vi "Omniax_mDrive_Zonly_2019EPICS.vi"() -> ()   [LabVIEW 2015]
uses:
  <vilib>/Utility/file.llb/Read From Spreadsheet File (I64).vi
  <vilib>/Utility/file.llb/Read From Spreadsheet File (string).vi
  <userlib>/caLab/Private/Put_DBL_PV.vi
  <vilib>/Instr/_visa.llb/VISA Configure Serial Port (Instr).vi
  <userlib>/caLab/Private/Get_PV.vi
  <userlib>/caLab/Private/Put_DBL-1D_PV-1D.vi
  <userlib>/caLab/Private/Get_PV-1D.vi
  <vilib>/Utility/file.llb/Write To Spreadsheet File (I64).vi
panel:
  out "x = y?":bool
  out "EPICS RQs":dbl[][](array[numeric])
  out "Status":bool
  in  "Pressure Overide":bool
  in  "Crash Override":bool
  in  "Open?":bool
  in  "Facing up?":bool
  in  "Heater retracted?":bool
  out "APX:MZ_MVG":bool
  out "inside HPC?":bool
  out "HPC01<0.001?":bool
  out "APX:V5 opened?":bool
  out "Isolated from GND?":bool
  out "APX:MZ_LIM":bool
  out "APX:MZ_RDY":bool
  in  "APX:MZ_RQ":dbl=10.0 min=10.0 max=60.0 step=0.1 format="%_6g"
  in  "APX:MZ_VLC_RQ":dbl=0.40000000000000013 min=0.1 max=0.61 step=0.1
  out "Z Velocity SP step/sec":i32=102400 min=1 max=153600
  out "Z Step SP":i32=-20000 min=0 max=102400000 step=500
  out "Z Step PV":i32 max=2000
  out "Dev5 Voltage":dbl
  out "Z max step":i32
  in  "V5 position 15360000":i32
  out "APX:MZ_VLC_PV":dbl format="%.3f"
  out "Presets":i32[][](array[numeric])
  in  "stop":bool
  in  "Tab Control 3":enum32{"Console", "Reset", "Bypass"}(tab)
  out "APX:MZ status":string="Cancel"
  out "Status Message":string="HP cell pressure too high! or "
  in  "Reset Z Position mm":dbl
  out "Reset Z Motor Steps":i32
  in  "Reset":bool
  out "Z Position MV mm":dbl
  in  "Clear ZY":bool
  out "R Backlash steps/sec":i32
  out "R Backlash":i32
  out "R Holding Current %":i32
  out "R Run Current %":i32
  out "R offset deg":dbl
  out "R deg/rev":dbl
  out "R steps/rev":u32
  out "R velocity PV step/sec":i32
  out "Z COM PORT":refnum<visa-resource-name>="COM5"
  out "Z Backlash steps/sec":i32
  out "Z Backlash":i32
  out "Z Holding Current %":i32
  out "Z Run Current %":i32
  out "Z offset mm":dbl
  out "Z mm/rev":dbl
  out "Z steps/rev":u32
  out "Z  velocity PV step/sec":i32=102400
  out "Z MINPOS":i32=-94296
  out "Z MAXPOS":i32=-34296
  out "APX:MZ_PV":dbl format="%_5g"
  out "X velocity PV step/sec":i32
  out "X Backlash steps/sec":i32
  out "X Backlash":i32
  out "X Holding Current %":i32
  out "X Run Current %":i32
  out "X offset mm":dbl
  out "X mm/rev":dbl
  out "X steps/rev":u32
  out "Y Backlash steps/sec":i32
  out "Y Backlash":i32
  out "Y Holding Current %":i32
  out "Y Run Current %":i32
  out "Y offset mm":dbl
  out "Y mm/rev":dbl
  out "Y steps/rev":u32
  out "Y velocity PV step/sec":i32
  in  "APX:MXYZR_STOP":bool
  # "COM14"
  # "APX:MZ"
  # "355.7"
  # "345"
  # "20 degree"
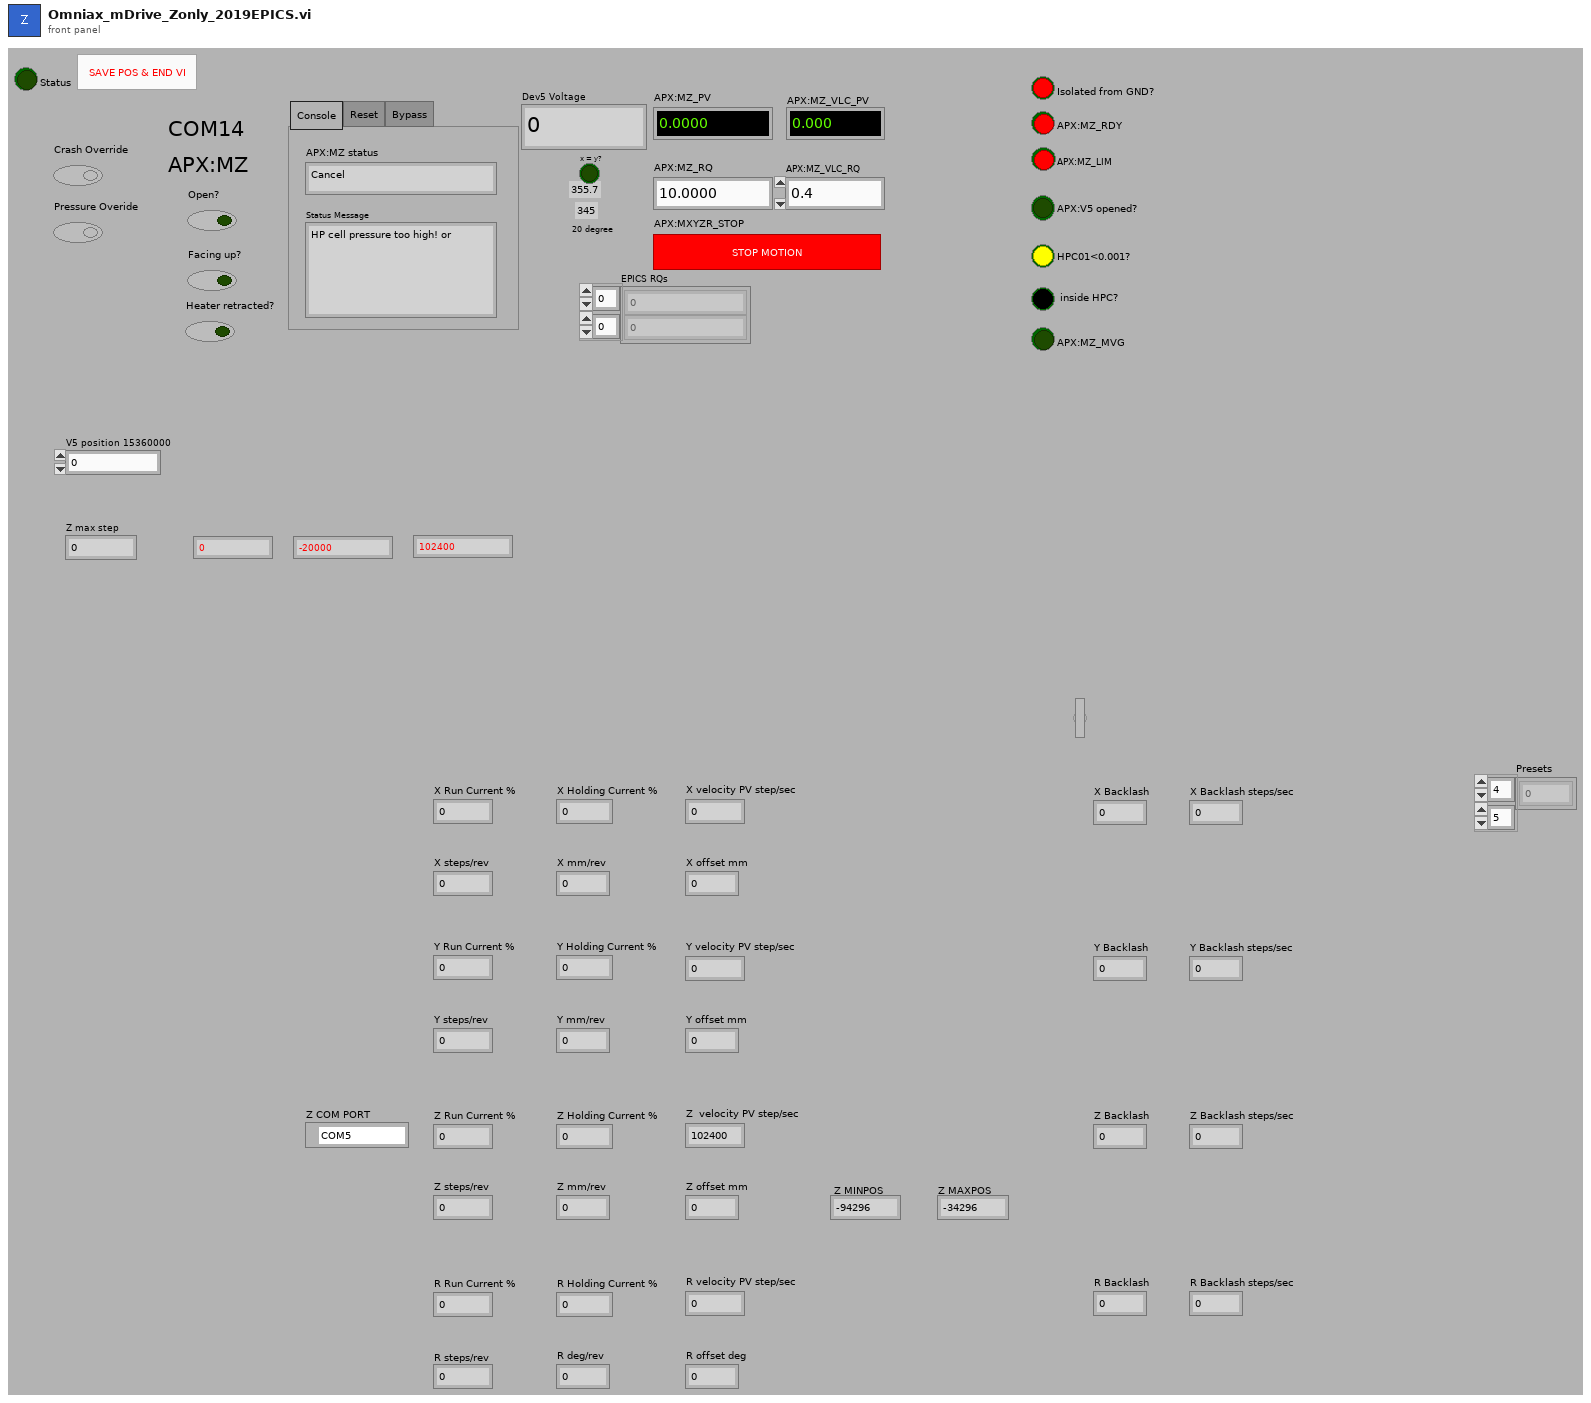
[diagram p1: front panel]
types:
  T1 = enum16{"Stop", "Reset", "Run Current", "Holding Current", "Accel Rate", "Decel Rate", "Move to Relative Position", "Move to Absolute Position", "Echo Mode", "Print Parameter", "Send String", "Microstep Resolution", "Set Current Position", "Max Velocity"}
  T2 = enum8{"Enabled", "Disabled", "Disabled and Grayed Out"}
  T3 = cluster{"first row[0]":i64, "first row[1]":i64, "first row[2]":i64, "first row[3]":i64, "first row[4]":i64, "first row[5]":i64, "first row[6]":i64, "first row[7]":i64, "first row[8]":i64}
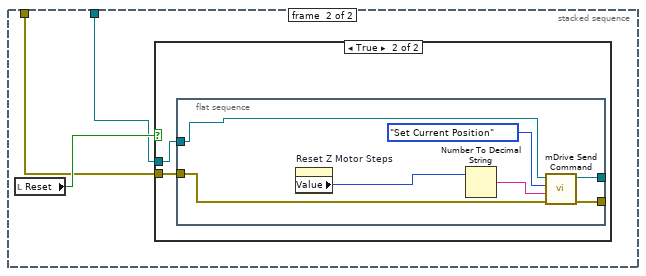
[diagram p4: hidden frame]
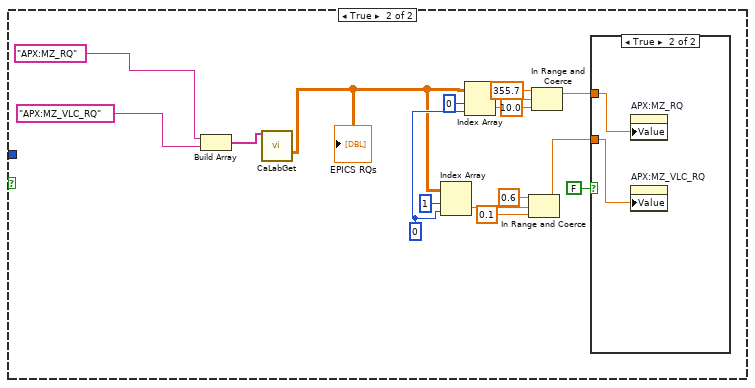
[diagram p7: hidden frame]
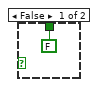
[diagram p9: hidden frame]
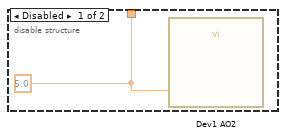
[diagram p10: hidden frame]
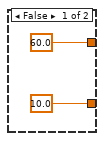
[diagram p12: hidden frame]
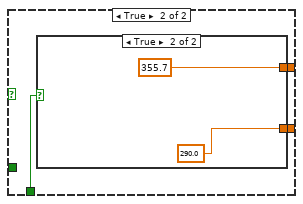
[diagram p13: hidden frame]
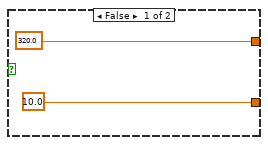
[diagram p14: hidden frame]
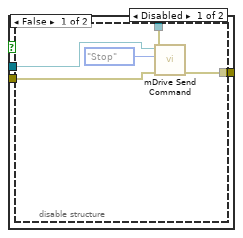
[diagram p15: hidden frame]
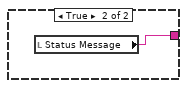
[diagram p17: hidden frame]
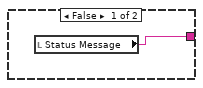
[diagram p18: hidden frame]
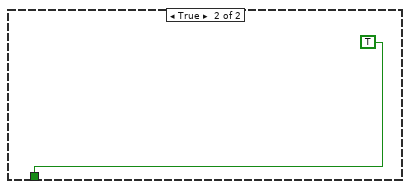
[diagram p19: hidden frame]
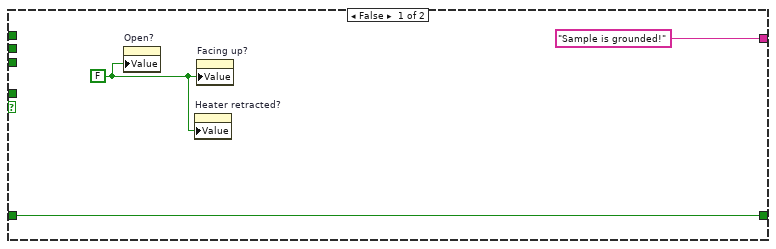
[diagram p20: hidden frame]
diagram:
  w4 = 0 ("dimension size")
  (unwired) 6144000 ("upper limit")
  (unwired) -6144000 ("lower limit")
  n1 = flat-sequence {
    tunnel: [w41] -> w23
    tunnel: [w42] -> w22
    tunnel: w23 -> [w57]
    tunnel: w22 -> [w56]
    tunnel: [w54] -> w2
    tunnel: [w52] -> w1
    tunnel: [w64] -> w27
    tunnel: [w60] -> w26
    tunnel: w2 -> [w61]
    tunnel: w1 -> [w60]
    tunnel: [w71] -> w38
    tunnel: [w73] -> w37
    tunnel: w27 -> [w72]
    tunnel: w26 -> [w74]
    tunnel: w38 -> [w81]
    tunnel: [w80] -> w36
    tunnel: w37 -> [w78]
    tunnel: [w79] -> w35
    tunnel: [w91] -> w34
    tunnel: [w92] -> w33
    tunnel: w36 -> [w90]
    tunnel: w35 -> [w89]
    tunnel: w34 -> [w102]
    tunnel: w33 -> [w101]
    tunnel: [w104] -> w32
    tunnel: [w103] -> w31
    tunnel: [w98] -> w30
    tunnel: [w111] -> w28
    tunnel: [w112] -> w29
    tunnel: w32 -> [w112]
    tunnel: w31 -> [w111]
    tunnel: w30 -> [w109]
    frame #0 {
      n2 = call-poly <userlib>:"CaLabPut.vi"("Value"=1.0, "PV Name"="SES:CalOff_RQ") -> ()  [unwired: 6 in, 4 out]
    }
    frame #1 {
      w49 = refnum<visa-resource-name> "COM14" ("COM PORT")
      w47 = u16 0 items=["None", "XON/XOFF", "RTS/CTS", "XON/XOFF & RTS/CTS", "DTR/DSR", "XON/XOFF & DTR/DSR"] ("flow control (0:none)")
      w46 = u16 10 items=["1.0"=10, "1.5"=15, "2.0"=20] ("stop bits (10: 1 bit)")
      # "Stop bits"
      n3 = call-poly "VISA Configure Serial Port"("VISA resource name"=w49, "timeout (10sec)"=u32 10000, "baud rate (9600)"=u32 9600, "data bits (8)"=u16 8, "parity (0:none)"=enum16{"None", "Odd", "Even", "Mark", "Space"}."None", "stop bits (10: 1 bit)"=w46, "flow control (0:none)"=w47) -> ("VISA resource name out"=w41:refnum<visa-resource-name>, "error out"=w42:errorcluster)  [unwired: 7 in]
      "Z COM PORT" <- w49
    }
    frame #2 {
      n4 = call "mDrive Send Command.vi"("error in (no error)"=w56, "Extra"="EM 2", "Command"=T1."Send String", "VISA resource name"=w57) -> ("error out"=w53:errorcluster, "VISA resource name out"=w55:refnum<visa-resource-name>)  [unwired: 3 in, 1 out]
      n5 = call "mDrive Send Command.vi"("error in (no error)"=w53, "Extra"="PR EE", "Command"=T1."Send String", "VISA resource name"=w55) -> ("error out"=w52:errorcluster, "VISA resource name out"=w54:refnum<visa-resource-name>)  [unwired: 3 in, 1 out]
    }
    frame #3 {
      n6 = Number To Decimal String(number=1000000) -> (decimal integer string=w62:string)  [unwired: 1 in]
      n7 = call "mDrive Send Command.vi"("Extra"=w62, "Command"=T1."Accel Rate", "VISA resource name"=w61) -> ("VISA resource name out"=w67:refnum<visa-resource-name>)  [unwired: 4 in, 2 out]
      n8 = call "mDrive Send Command.vi"("Extra"=w62, "Command"=T1."Decel Rate", "VISA resource name"=w67) -> ("VISA resource name out"=w64:refnum<visa-resource-name>)  [unwired: 4 in, 2 out]
    }
    frame #4 {
      # "Run Current %"
      n9 = property on="Z Run Current %" class="DigNum (strict)"() -> ("Value"=w69:i32)  [unwired: 2 in, 2 out]
      n10 = Number To Decimal String(number=w69) -> (decimal integer string=w70:string)  [unwired: 1 in]
      n11 = call "mDrive Send Command.vi"("error in (no error)"=w74, "Extra"=w70, "Command"=T1."Run Current", "VISA resource name"=w72) -> ("error out"=w73:errorcluster, "VISA resource name out"=w71:refnum<visa-resource-name>)  [unwired: 3 in, 1 out]
    }
    frame #5 {
      # "Holding Current %"
      n12 = property on="Z Run Current %" class="DigNum (strict)"() -> ("Value"=w76:i32)  [unwired: 2 in, 2 out]
      n13 = Number To Decimal String(number=w76) -> (decimal integer string=w77:string)  [unwired: 1 in]
      n14 = call "mDrive Send Command.vi"("error in (no error)"=w78, "Extra"=w77, "Command"=T1."Holding Current", "VISA resource name"=w81) -> ("error out"=w79:errorcluster, "VISA resource name out"=w80:refnum<visa-resource-name>)  [unwired: 3 in, 1 out]
    }
    frame #6 {
      # "Velocity Max"
      n15 = property on="Z Velocity SP step/sec" class="DigNum (strict)"() -> ("Value"=w88:i32)  [unwired: 2 in, 2 out]
      n16 = Number To Decimal String(number=w88) -> (decimal integer string=w87:string)  [unwired: 1 in]
      n17 = call "mDrive Send Command.vi"("error in (no error)"=w89, "Extra"=w87, "Command"=T1."Max Velocity", "VISA resource name"=w90) -> ("error out"=w85:errorcluster, "VISA resource name out"=w95:refnum<visa-resource-name>)  [unwired: 3 in, 1 out]
      n18 = call "mDrive Send Command.vi"("error in (no error)"=w85, "Extra"="VM", "Command"=T1."Print Parameter", "VISA resource name"=w95) -> ("error out"=w92:errorcluster, "read buffer"=w93:string, "VISA resource name out"=w91:refnum<visa-resource-name>)  [unwired: 3 in]
      n19 = Decimal String To Number(string=w93, offset=0) -> (number=w86:i32)  [unwired: 1 in, 1 out]
      n20 = property on="Z  velocity PV step/sec" class="DigNum (strict)"("Val(Sgnl)"=w86) -> ()  [unwired: 2 in, 2 out]
    }
    frame #7 {
      # "PRINT POSITION"
      n21 = call "mDrive Send Command.vi"("error in (no error)"=w101, "Extra"="P", "Command"=T1."Print Parameter", "VISA resource name"=w102) -> ("error out"=w103:errorcluster, "read buffer"=w100:string, "VISA resource name out"=w104:refnum<visa-resource-name>)  [unwired: 3 in]
      n22 = Decimal String To Number(string=w100, offset=0) -> (number=w98:i32)  [unwired: 1 in, 1 out]
    }
    frame #8 {
      n23 = property on="Z Step SP" class="DigNum (strict)"("Val(Sgnl)"=w109) -> ()  [unwired: 2 in, 2 out]
      n24 = property on="Z Step SP" class="DigNum (strict)"() -> ("Maximum"=w106:dbl)  [unwired: 2 in, 2 out]
      n25 = property on="Z Step SP" class="DigNum (strict)"() -> ("Minimum"=w108:dbl)  [unwired: 2 in, 2 out]
      n26 = To Long Integer(number=w106) -> (32bit integer=w107:i32)
      "Z MAXPOS" <- w107
      n27 = To Long Integer(number=w108) -> (32bit integer=w105:i32)
      "Z MINPOS" <- w105
      n28 = In Range and Coerce(upper limit=w107, x=w109, lower limit=w105) -> (In Range?=w110:bool)  [unwired: 1 out]
      n29 = property on="APX:MZ_LIM" class="Bool (strict)"("Val(Sgnl)"=w110) -> ()  [unwired: 2 in, 2 out]
    }
  }
  n30 = flat-sequence {
    frame #0 {
      (unwired) 1.0 ("Data Entry Limits:Minimum")
      w116 = -3.0 ("R deg/rev")
      w114 = u32 51200 ("step/rev")
      n31 = To Double Precision Float(number=w114) -> (double precision float=w115:dbl)
      n32 = To Double Precision Float(number=10000 ("Value (Signaling)")) -> (double precision float=w120:dbl)
      n33 = Divide(x=w120, y=w115) -> (x/y=w119:dbl)
      n34 = Multiply(x=w119, y=w116) -> (x*y=w117:dbl)
      n35 = Absolute Value(x=w117) -> ()  [unwired: 1 out]
      "R offset deg" <- 0.0 ("R offset deg")
      "R deg/rev" <- w116
      "R steps/rev" <- w114
    }
  }
  n36 = flat-sequence {
    frame #0 {
      w123 = 0.2 ("Z mm/rev")
      w122 = u32 51200 ("step/rev")
      n37 = To Double Precision Float(number=153600 ("Value (Signaling)")) -> (double precision float=w128:dbl)
      n38 = To Double Precision Float(number=w122) -> (double precision float=w127:dbl)
      n39 = property on="Z Velocity SP step/sec" class="DigNum (strict)"("Val(Sgnl)"=51200 ("Value (Signaling)")) -> ()  [unwired: 2 in, 2 out]
      n40 = property on="Z Velocity SP step/sec" class="DigNum (strict)"("Minimum"=1.0 ("Data Entry Limits:Minimum")) -> ()  [unwired: 2 in, 2 out]
      n41 = Divide(x=w128, y=w127) -> (x/y=w125:dbl)
      n42 = property on="Z Velocity SP step/sec" class="DigNum (strict)"("Maximum"=w128) -> ()  [unwired: 2 in, 2 out]
      n43 = Multiply(x=w125, y=w123) -> (x*y=w126:dbl)
      n44 = property on="APX:MZ_VLC_RQ" class="DigNum (strict)"("Val(Sgnl)"=w126) -> ()  [unwired: 2 in, 2 out]
      "Z offset mm" <- 0.0 ("Z offset mm")
      "Z mm/rev" <- w123
      "Z steps/rev" <- w122
    }
  }
  n45 = disable-structure shown="Disabled" {
    frame Disabled {
      n46 = flat-sequence {
        frame #0 {
          w131 = FALSE ("Value (Signaling)")
          w134 = FALSE ("Value (Signaling)")
          w137 = FALSE ("Value (Signaling)")
          w138 = FALSE ("Value (Signaling)")
          "Z Backlash steps/sec" <- 25600 ("Z Backlash steps/sec")
          "Z Backlash" <- -51200 ("Z Backlash")
          "X Backlash steps/sec" <- 25600 ("Value (Signaling)")
          "X Backlash" <- 10240 ("Backlash2")
          "Y Backlash" <- -10240 ("Backlash2")
          "Y Backlash steps/sec" <- 25600 ("Value (Signaling)")
          "R Backlash steps/sec" <- 6400 ("R Backlash steps/sec")
          "R Backlash" <- -12800 ("R Backlash")
        }
      }
    }
    frame Enabled {
    }
  }
  n47 = flat-sequence {
    frame #0 {
      "Z Holding Current %" <- 20 ("Z Holding Current %")
      "Z Run Current %" <- 40 ("Z Run Current %")
      "X Run Current %" <- 40 ("Run Current %")
      "X Holding Current %" <- 20 ("Holding Current %")
      "Y Run Current %" <- 40 ("Run Current %")
      "Y Holding Current %" <- 20 ("Holding Current %")
      "R Holding Current %" <- 15 ("R Holding Current %")
      "R Run Current %" <- 80 ("R Run Current %")
    }
  }
  n48 = flat-sequence {
    frame #0 {
      (unwired) 0.1 ("Value (Signaling)")
      (unwired) FALSE ("Value (Signaling)")
      (unwired) T2."Disabled and Grayed Out" ("Disabled")
      (unwired) T2."Disabled and Grayed Out" ("Disabled")
      (unwired) 0.1 ("Value (Signaling)")
      (unwired) FALSE ("Value (Signaling)")
      (unwired) 0.1 ("Value (Signaling)")
      (unwired) FALSE ("Value (Signaling)")
      (unwired) 0.1 ("Value (Signaling)")
      (unwired) FALSE ("Value (Signaling)")
    }
  }
  n49 = flat-sequence {
    frame #0 {
      w153 = 0.2 ("MM/rev")
      w155 = u32 51200 ("step/rev")
      (unwired) 1.0 ("Data Entry Limits:Minimum")
      # "a=1000000"
      n50 = To Double Precision Float(number=128000 ("Value (Signaling)")) -> (double precision float=w156:dbl)
      n51 = To Double Precision Float(number=w155) -> (double precision float=w154:dbl)
      n52 = Divide(x=w156, y=w154) -> (x/y=w152:dbl)
      n53 = Multiply(x=w152, y=w153) -> ()  [unwired: 1 out]
      "X offset mm" <- 0.0 ("offset")
      "X steps/rev" <- w155
      "X mm/rev" <- w153
    }
  }
  n54 = flat-sequence {
    frame #0 {
      w160 = 0.2 ("MM/rev")
      w162 = u32 51200 ("step/rev")
      (unwired) 1.0 ("Data Entry Limits:Minimum")
      n55 = To Double Precision Float(number=128000 ("Value (Signaling)")) -> (double precision float=w163:dbl)
      n56 = To Double Precision Float(number=w162) -> (double precision float=w161:dbl)
      n57 = Divide(x=w163, y=w161) -> (x/y=w159:dbl)
      n58 = Multiply(x=w159, y=w160) -> ()  [unwired: 1 out]
      "Y offset mm" <- 0.0 ("offset")
      "Y steps/rev" <- w162
      "Y mm/rev" <- w160
    }
  }
  n59 = property on="Z Step SP" class="DigNum (strict)"("Minimum"=0 ("lower limit")) -> ()  [unwired: 2 in, 2 out]
  n60 = property on="V5 position 15360000" class="DigNum (strict)"("Value"=15360000 ("V5 position 15360000")) -> ()  [unwired: 2 in, 2 out]
  n61 = property on="Z Step SP" class="DigNum (strict)"("Maximum"=102400000 ("upper limit")) -> ()  [unwired: 2 in, 2 out]
  n62 = call-poly <vilib>:"Read From Spreadsheet File.vi"("file path (dialog if empty)"=path "S:/SSE/IMS/POSZ.TXT") -> ("first row"=w18:i64[])  [unwired: 6 in, 4 out]
  n63 = call-poly <vilib>:"Read From Spreadsheet File.vi"("file path (dialog if empty)"=path "S:/SSE/IMS/PRESET.TXT") -> ("all rows"=w10:string[][])  [unwired: 6 in, 4 out]
  n64 = Array To Cluster(array=w18) -> (cluster=w17:T3)
  n65 = Transpose 2D Array(2D array=w10) -> (transposed array=w11:string[][])
  n66 = Unbundle(w17) -> ("first row[2]"=w15:i64)  [unwired: 8 out]
  n67 = Delete From Array(array=w11, index (row)=0) -> (array with subset deleted=w13:string[][])  [unwired: 2 in, 1 out]
  n68 = property on="Reset Z Motor Steps" class="DigNum (strict)"("Val(Sgnl)"=w15) -> ()  [unwired: 2 in, 2 out]
  n69 = Transpose 2D Array(2D array=w13) -> (transposed array=w14:string[][])
  n70 = Decimal String To Number(string=w14) -> (number=w12:i32[][])  [unwired: 2 in, 1 out]
  n71 = Initialize Array(w4, w4, 4 ("dimension size")) -> (w7:i32[][])
  n72 = Build Array (concatenate)(w7, w12) -> (→"Presets":i32[][])
  n73 = while {
    tunnel: w29 -> [w171]
    tunnel: w28 -> [w170]
    tunnel: [w180] -> w21
    tunnel: [w179] -> w20
    i -> [w172]
    stop <- "stop" stop-if-true
    n74 = Quotient & Remainder(x=w172, y=2) -> (x-y*floor(x/y)=w176:i32)  [unwired: 1 out]
    n75 = Greater?(x=w172, y=2.0) -> (0:w173:bool)
    n76 = Equal To 0?(x=w176) -> (x = 0?=w177:bool)
    n77 = case shown="True" w177 {
      tunnel: [FALSE ("Status") TRUE ("Status")] -> w169
      frame False {
      }
      frame True {
      }
    }
    "Status" <- w169
    n78 = case shown="False" w173 {
      tunnel: w172 -> [w231 _]
      frame False {
        n79 = Equal?(x=w231, y=0.0) -> (x = y?=w230:bool)
        n80 = case shown="True" w230 {
          frame False {
          }
          frame True {
            n81 = local read "APX:MZ_VLC_PV"() -> (w233:dbl)
            n82 = local read "APX:MZ_PV"() -> (w234:dbl)
            n83 = Build Array("APX:MZ_RQ", "APX:MZ_VLC_RQ") -> (w236:string[])
            n84 = Build Array(w234, w233) -> (w235:dbl[])
            n85 = call-poly <userlib>:"CaLabPut.vi"("Values"=w235, "PV Names"=w236) -> ()  [unwired: 6 in, 4 out]
          }
        }
      }
      frame True {
        w249 = 0 ("index (col)")
        n86 = Build Array("APX:MZ_RQ", "APX:MZ_VLC_RQ") -> (w254:string[])
        n87 = call-poly "CaLabGet.vi"("PV Names"=w254) -> ("Value Array (number)"=w248:dbl[][])  [unwired: 8 in, 6 out]
        "EPICS RQs" <- w248
        n88 = Index Array(array=w248, index (row)=1, index (col)=w249) -> (element=w247:dbl)
        n89 = Index Array(array=w248, index (row)=0, index (col)=w249) -> (element=w244:dbl)
        n90 = In Range and Coerce(upper limit=0.6, x=w247, lower limit=0.1) -> (coerced(x)=w239:dbl)  [unwired: 1 out]
        n91 = In Range and Coerce(upper limit=355.7, x=w244, lower limit=10.0) -> (coerced(x)=w240:dbl)  [unwired: 1 out]
        n92 = case shown="True" FALSE {
          tunnel: w240 -> [_ w255]
          tunnel: w239 -> [_ w256]
          frame False {
          }
          frame True {
            n93 = property on="APX:MZ_RQ" class="DigNum (strict)"("Value"=w255) -> ()  [unwired: 2 in, 2 out]
            n94 = property on="APX:MZ_VLC_RQ" class="DigNum (strict)"("Value"=w256) -> ()  [unwired: 2 in, 2 out]
          }
        }
      }
    }
    n95 = flat-sequence {
      frame #0 {
        n96 = property on="Reset Z Position mm" class="DigNum (strict)"() -> ("Value"=w184:dbl)  [unwired: 2 in, 2 out]
        n97 = property on="Z offset mm" class="DigNum (strict)"() -> ("Value"=w192:dbl)  [unwired: 2 in, 2 out]
        n98 = Subtract(x=w184, y=w192) -> (x-y=w185:dbl)
        n99 = property on="Z steps/rev" class="DigNum (strict)"() -> ("Value"=w190:u32)  [unwired: 2 in, 2 out]
        n100 = property on="Z mm/rev" class="DigNum (strict)"() -> ("Value"=w191:dbl)  [unwired: 2 in, 2 out]
        n101 = Divide(x=w185, y=w191) -> (x/y=w186:dbl)
        n102 = To Double Precision Float(number=w190) -> (double precision float=w187:dbl)
        n103 = Multiply(x=w186, y=w187) -> (x*y=w188:dbl)
        n104 = To Long Integer(number=w188) -> (32bit integer=w189:i32)
        n105 = property on="Reset Z Motor Steps" class="DigNum (strict)"("Val(Sgnl)"=w189) -> ()  [unwired: 2 in, 2 out]
      }
      frame #1 {
        n106 = property on="Z steps/rev" class="DigNum (strict)"() -> ("Value"=w205:u32)  [unwired: 2 in, 2 out]
        n107 = property on="Z steps/rev" class="DigNum (strict)"() -> ("Value"=w198:u32)  [unwired: 2 in, 2 out]
        n108 = property on="Z Velocity SP step/sec" class="DigNum (strict)"() -> ("Value"=w196:i32)  [unwired: 2 in, 2 out]
        n109 = property on="Z Step SP" class="DigNum (strict)"() -> ("Value"=w203:i32)  [unwired: 2 in, 2 out]
        n110 = To Double Precision Float(number=w203) -> (double precision float=w202:dbl)
        n111 = To Double Precision Float(number=w205) -> (double precision float=w199:dbl)
        n112 = To Double Precision Float(number=w196) -> (double precision float=w195:dbl)
        n113 = To Double Precision Float(number=w198) -> (double precision float=w193:dbl)
        n114 = Divide(x=w202, y=w199) -> (x/y=w200:dbl)
        n115 = Divide(x=w195, y=w193) -> (x/y=w194:dbl)
        n116 = property on="Z mm/rev" class="DigNum (strict)"() -> ("Value"=w207:dbl)  [unwired: 2 in, 2 out]
        n117 = property on="Z offset mm" class="DigNum (strict)"() -> ("Value"=w206:dbl)  [unwired: 2 in, 2 out]
        n118 = Multiply(x=w200, y=w207) -> (x*y=w201:dbl)
        n119 = Multiply(x=w194, y=w207) -> (x*y=w197:dbl)
        n120 = property on="APX:MZ_VLC_PV" class="DigNum (strict)"("Val(Sgnl)"=w197) -> ()  [unwired: 2 in, 2 out]
        n121 = Add(x=w201, y=w206) -> (x+y=w204:dbl)
        n122 = property on="Z Position MV mm" class="DigNum (strict)"("Val(Sgnl)"=w204) -> ()  [unwired: 2 in, 2 out]
      }
    }
    n123 = stacked-sequence {
      tunnel: w171 -> [w209 w219]
      tunnel: w170 -> [w208 w218]
      frame #0 {
        n124 = local read "APX:MXYZR_STOP"() -> (w210:bool)
        n125 = case shown="True" w210 {
          tunnel: w209 -> [_ w212]
          tunnel: w208 -> [_ w211]
          frame False {
          }
          frame True {
            n126 = flat-sequence {
              tunnel: [w216] -> _
              tunnel: [w215] -> _
              tunnel: w212 -> [w214]
              tunnel: w211 -> [w213]
              frame #0 {
                n127 = call "mDrive Send Command.vi"("error in (no error)"=w213, "Command"=T1."Stop", "VISA resource name"=w214) -> ("error out"=w215:errorcluster, "VISA resource name out"=w216:refnum<visa-resource-name>)  [unwired: 4 in, 1 out]
              }
            }
          }
        }
      }
      frame #1 {
        n128 = local read "Reset"() -> (w220:bool)
        n129 = case shown="True" w220 {
          tunnel: w219 -> [_ w222]
          tunnel: w218 -> [_ w221]
          frame False {
          }
          frame True {
            n130 = flat-sequence {
              tunnel: [w226] -> _
              tunnel: [w225] -> _
              tunnel: w222 -> [w224]
              tunnel: w221 -> [w223]
              frame #0 {
                n131 = property on="Reset Z Motor Steps" class="DigNum (strict)"() -> ("Value"=w227:i32)  [unwired: 2 in, 2 out]
                n132 = Number To Decimal String(number=w227) -> (decimal integer string=w228:string)  [unwired: 1 in]
                n133 = call "mDrive Send Command.vi"("error in (no error)"=w223, "Extra"=w228, "Command"=T1."Set Current Position", "VISA resource name"=w224) -> ("error out"=w225:errorcluster, "VISA resource name out"=w226:refnum<visa-resource-name>)  [unwired: 3 in, 1 out]
              }
            }
          }
        }
      }
    }
    n134 = local read "APX:MZ_RQ"() -> (w168:dbl)
    n135 = flat-sequence {
      tunnel: ["APX:MZ_RQ"] -> w167
      tunnel: [w182] -> _
      tunnel: w168 -> [w182]
      tunnel: [w182] -> w166
      frame #0 {
      }
    }
    n136 = Equal?(x=w167, y=w166) -> (x = y?=→"x = y?":bool)
    n137 = event shown="[0] Timeout" {
      selector: _ -> [_ _]
      dyn-events: _ -> [_ _]
      timeout: 200 -> [_ _]
      tunnel: w171 -> [w280 w557]
      tunnel: w170 -> [w281 w556]
      tunnel: [w296 w554] -> w180
      tunnel: [w295 w555] -> w179
      event Timeout {
        n138 = event-data() -> ()  [unwired: 1 in, 2 out]
        n139 = flat-sequence {
          tunnel: [w348] -> w277
          frame #0 {
            n140 = case shown="False" "Pressure Overide" {
              tunnel: [w353 TRUE] -> w348
              frame False {
                n141 = call-poly "CaLabGet.vi"("PV Name"="APX:HPC01") -> ("1rst Value (number)"=w359:dbl, "Error out"=w356:errorcluster)  [unwired: 8 in, 5 out]
                n142 = call-poly "CaLabGet.vi"("PV Name"="APX:V5_SOP", "Error in (no error)"=w356) -> ("1rst Value (number)"=w355:dbl)  [unwired: 7 in, 6 out]
                n143 = Less?(x=w359, y=0.001) -> (x < y?=w352:bool)
                "HPC01<0.001?" <- w352
                n144 = Number To Boolean Array(number=w355) -> (Boolean array=w354:bool[])
                n145 = case shown="True" w352 {
                  tunnel: [w363 "HP cell pressure too high!"] -> w351
                  frame False {
                    n146 = local read "Status Message"() -> (w363:string)
                  }
                  frame True {
                  }
                }
                n147 = Index Array(array=w354) -> (element=w349:bool)  [unwired: 1 in]
                "APX:V5 opened?" <- w349
                n148 = case shown="False" w349 {
                  tunnel: ["HP Turbo GV is closed." w362] -> w350
                  frame False {
                  }
                  frame True {
                    n149 = local read "Status Message"() -> (w362:string)
                  }
                }
                n150 = Or(x=w352, y=w349) -> (x .or. y?=w353:bool)
                n151 = local write "Status Message"(w351) -> ()
                n152 = local write "Status Message"(w350) -> ()
              }
              frame True {
              }
            }
          }
        }
        n153 = property on="Open?" class="Bool (strict)"() -> ("Value"=w265:bool)  [unwired: 2 in, 2 out]
        n154 = property on="Facing up?" class="Bool (strict)"() -> ("Value"=w266:bool)  [unwired: 2 in, 2 out]
        n155 = property on="Facing up?" class="Bool (strict)"() -> ("Value"=w275:bool)  [unwired: 2 in, 2 out]
        n156 = property on="Heater retracted?" class="Bool (strict)"() -> ("Value"=w267:bool)  [unwired: 2 in, 2 out]
        n157 = property on="Isolated from GND?" class="Bool (strict)"() -> ("Value"=w285:bool)  [unwired: 2 in, 2 out]
        n158 = property on="Heater retracted?" class="Bool (strict)"() -> ("Value"=w276:bool)  [unwired: 2 in, 2 out]
        n159 = And(x=w266, y=w267) -> (x .and. y?=w264:bool)
        n160 = And(x=w265, y=w264) -> (x .and. y?=w263:bool)
        n161 = case shown="True" w263 {
          tunnel: [w419 w420] -> w294
          frame False {
            n162 = property on="V5 position 15360000" class="DigNum (strict)"() -> ("Value"=w419:i32)  [unwired: 2 in, 2 out]
          }
          frame True {
            n163 = property on="Z Step SP" class="DigNum (strict)"() -> ("Maximum"=w420:dbl)  [unwired: 2 in, 2 out]
          }
        }
        "Z max step" <- w294
        n164 = property on="Open?" class="Bool (strict)"() -> ("Value"=w282:bool)  [unwired: 2 in, 2 out]
        n165 = And(x=w275, y=w276) -> (x .and. y?=w274:bool)
        n166 = property on="APX:MZ_PV" class="DigNum (strict)"() -> ("Value"=w269:dbl)  [unwired: 2 in, 2 out]
        n167 = And(x=w282, y=w274) -> (x .and. y?=w289:bool)
        n168 = property on="inside HPC?" class="Bool (strict)"() -> ("Value"=w283:bool)  [unwired: 2 in, 2 out]
        n169 = call-poly <userlib>:"CaLabPut.vi"("Value"=w269, "PV Name"="APX:OmniaxZ") -> ()  [unwired: 6 in, 4 out]
        n170 = Greater Or Equal?(x=w269, y=320.0) -> (x >= y?=w268:bool)
        n171 = And(x=w285, y=w289) -> (x .and. y?=w262:bool)
        n172 = Greater?(x=w269, y=55.0) -> (0:w290:bool)
        n173 = Greater?(x=w269, y=289.0) -> (0:w273:bool)
        n174 = flat-sequence {
          frame #0 {
            w308 = 10 ("number of samples")
            # "ai16 p0.16"
            # "Crash Sensing"
            n175 = call "Dev1 AI0"("number of samples"=w308) -> ("data"=w313:dynamicdata)  [unwired: 16 in, 2 out]
            n176 = call "Convert from Dynamic Data"("Dynamic Data Type"=w313) -> ("Array"=w314:dbl[])  [unwired: 3 in]
            n177 = disable-structure shown="Enabled" {
              disable-tunnel: [w320 5.0 ("data")] -> w319
              frame Disabled {
                w320 = 5.0 ("data")
                n178 = call "Dev1 AO2"("data"=w320) -> ()  [unwired: 17 in, 2 out]
              }
              frame Enabled {
                n179 = call "Dev1 P1.7"("data"=bool[] [TRUE]) -> ()  [unwired: 17 in, 2 out]
              }
            }
            n180 = Add Array Elements(numeric array=w314) -> (sum=w312:dbl)
            n181 = Divide(x=w312, y=w308) -> (x/y=w311:dbl)
            n182 = Absolute Value(x=w311) -> (abs(x)=w315:dbl)
            "Dev5 Voltage" <- w315
            n183 = Multiply(x=w319, y=0.8) -> (x*y=w309:dbl)
            n184 = Greater?(x=w315, y=w309) -> (0:w316:bool)
            n185 = case shown="True" "Crash Override" {
              tunnel: [w323 TRUE] -> w317
              tunnel: w316 -> [w323 _]
              frame False {
              }
              frame True {
              }
            }
            "Isolated from GND?" <- w317
          }
        }
        n186 = case shown="True" w290 {
          tunnel: w285 -> [w368 _]
          tunnel: [w368 w374] -> w278
          tunnel: w262 -> [_ w374]
          tunnel: ["Sample is grounded!" w372] -> w286
          tunnel: w273 -> [_ w373]
          tunnel: w283 -> [_ w371]
          tunnel: w282 -> [_ w370]
          tunnel: w275 -> [_ w369]
          frame False {
            w366 = FALSE ("Open?")
            n187 = property on="Open?" class="Bool (strict)"("Value"=w366) -> ()  [unwired: 2 in, 2 out]
            n188 = property on="Heater retracted?" class="Bool (strict)"("Value"=w366) -> ()  [unwired: 2 in, 2 out]
            n189 = property on="Facing up?" class="Bool (strict)"("Value"=w366) -> ()  [unwired: 2 in, 2 out]
          }
          frame True {
            n190 = case shown="True" w373 {
              tunnel: [w376 "Be careful, the sample enters into the HP cell!"] -> w372
              tunnel: w371 -> [_ w393]
              tunnel: w370 -> [w381 _]
              tunnel: w369 -> [w380 _]
              frame False {
                w377 = "\r"
                w376 = "Is the gate valve opened? Is the sample facing up?  Is the lamp heater retracted?"
                n191 = disable-structure shown="Disabled" {
                  disable-tunnel: w381 -> [w386 _]
                  disable-tunnel: w380 -> [w385 _]
                  disable-tunnel: [w384 _] -> w379
                  disable-tunnel: [w383 _] -> w378
                  frame Disabled {
                    n192 = case shown="True" w386 {
                      tunnel: ["Is the sample facing up?" ""] -> w384
                      frame False {
                      }
                      frame True {
                      }
                    }
                    n193 = case shown="True" w385 {
                      tunnel: ["Is the gate valve opened?" ""] -> w383
                      frame False {
                      }
                      frame True {
                      }
                    }
                  }
                  frame Enabled {
                  }
                }
                n194 = property on="inside HPC?" class="Bool (strict)"("Value"=FALSE ("inside HPC?")) -> ()  [unwired: 2 in, 2 out]
                n195 = Concatenate Strings(w379, w377, w378, w377, w376) -> (w375:string)
                n196 = local write "Status Message"(w375) -> ()
              }
              frame True {
                n197 = case shown="True" w393 {
                  frame False {
                  }
                  frame True {
                    n198 = local write "Status Message"("Sample is touching HPC!") -> ()
                  }
                }
                n199 = property on="APX:MZ_VLC_RQ" class="DigNum (strict)"("Value"=0.1 ("APX:MZ_VLC_RQ")) -> ()  [unwired: 2 in, 2 out]
                n200 = property on="inside HPC?" class="Bool (strict)"("Value"=TRUE ("inside HPC?")) -> ()  [unwired: 2 in, 2 out]
              }
            }
          }
        }
        n201 = case shown="True" w277 {
          tunnel: w281 -> [w341 w346]
          tunnel: [w340 w346] -> w279
          tunnel: w280 -> [w339 _]
          frame False {
            n202 = disable-structure shown="Disabled" {
              disable-tunnel: w341 -> [w344 _]
              disable-tunnel: [w343 _] -> w340
              disable-tunnel: w339 -> [w342 _]
              frame Disabled {
                n203 = call "mDrive Send Command.vi"("error in (no error)"=w344, "Command"=T1."Stop", "VISA resource name"=w342) -> ("error out"=w343:errorcluster)  [unwired: 4 in, 2 out]
              }
              frame Enabled {
              }
            }
          }
          frame True {
          }
        }
        n204 = Or(x=w277, y=w278) -> (x .or. y?=w261:bool)
        n205 = property on="Isolated from GND?" class="Bool (strict)"() -> ("Value"=w260:bool)  [unwired: 2 in, 2 out]
        n206 = case shown="False" w273 {
          tunnel: [w327 w334] -> w272
          tunnel: [w326 w333] -> w271
          tunnel: w268 -> [_ w332]
          tunnel: w262 -> [w325 _]
          frame False {
            n207 = case shown="True" w325 {
              tunnel: [60.0 ("Data Entry Limits:Maximum") 290.0 ("Data Entry Limits:Maximum")] -> w327
              tunnel: [10.0 ("Data Entry Limits:Minimum") 10.0 ("Data Entry Limits:Minimum")] -> w326
              frame False {
              }
              frame True {
              }
            }
          }
          frame True {
            n208 = case shown="True" w332 {
              tunnel: [320.0 ("Data Entry Limits:Maximum") 355.7 ("Data Entry Limits:Maximum")] -> w334
              tunnel: [10.0 ("Data Entry Limits:Minimum") 290.0 ("Data Entry Limits:Minimum")] -> w333
              frame False {
              }
              frame True {
              }
            }
          }
        }
        n209 = And(x=w261, y=w260) -> (x .and. y?=w259:bool)
        n210 = case shown="False" w259 {
          tunnel: w280 -> [w403 w416]
          tunnel: [w402 w416] -> w293
          tunnel: [w400 w413] -> w292
          tunnel: w286 -> [w399 _]
          tunnel: w285 -> [w398 _]
          tunnel: [w397 w415] -> w284
          tunnel: w283 -> [_ w414]
          tunnel: w279 -> [w396 w413]
          frame False {
            n211 = case shown="False" w398 {
              tunnel: w399 -> [w404 w406]
              tunnel: [w404 "Be careful!"] -> w397
              frame False {
              }
              frame True {
                n212 = disable-structure shown="Disabled" {
                  disable-tunnel: [w409 _] -> w407
                  disable-tunnel: w406 -> [w408 _]
                  frame Disabled {
                    n213 = Two Button Dialog(message=w408, 1:"Cancel" ("F button name (\"Cancel\")"), 2:"OK" ("T button name (\"OK\")")) -> (T button?=w409:bool)
                  }
                  frame Enabled {
                  }
                }
                n214 = disable-structure shown="Disabled" {
                  disable-tunnel: w407 -> [w412 _]
                  frame Disabled {
                    n215 = property on="Open?" class="Bool (strict)"("Value"=w412) -> ()  [unwired: 2 in, 2 out]
                    n216 = property on="inside HPC?" class="Bool (strict)"("Value"=w412) -> ()  [unwired: 2 in, 2 out]
                    n217 = property on="Facing up?" class="Bool (strict)"("Value"=w412) -> ()  [unwired: 2 in, 2 out]
                  }
                  frame Enabled {
                  }
                }
              }
            }
            n218 = call "mDrive Send Command.vi"("error in (no error)"=w396, "Command"=T1."Stop", "VISA resource name"=w403) -> ("error out"=w400:errorcluster, "VISA resource name out"=w402:refnum<visa-resource-name>)  [unwired: 4 in, 1 out]
          }
          frame True {
            n219 = case shown="False" w414 {
              tunnel: ["Normal" "In HPC! Be careful! "] -> w415
              frame False {
              }
              frame True {
              }
            }
          }
        }
        "APX:MZ status" <- w284
        n220 = property on="APX:MZ_RQ" class="DigNum (strict)"("Maximum"=w272) -> ()  [unwired: 2 in, 2 out]
        n221 = property on="APX:MZ_RQ" class="DigNum (strict)"("Minimum"=w271) -> ()  [unwired: 2 in, 2 out]
        n222 = flat-sequence {
          tunnel: [w458] -> w307
          tunnel: [w437] -> w306
          tunnel: [w448] -> w305
          tunnel: [w428] -> w304
          tunnel: w293 -> [w427]
          tunnel: w292 -> [w426]
          tunnel: w307 -> [w462]
          tunnel: [w462] -> w303
          tunnel: w306 -> [w461]
          tunnel: [w461] -> w302
          tunnel: w305 -> [w460]
          tunnel: [w460] -> w301
          tunnel: w304 -> [w459]
          tunnel: [w459] -> w300
          tunnel: w303 -> [w465]
          tunnel: [w466] -> w299
          tunnel: w302 -> [w468]
          tunnel: [w467] -> w298
          tunnel: w301 -> [w464]
          tunnel: [w463] -> w297
          tunnel: w300 -> [w463]
          tunnel: w299 -> [w478]
          tunnel: w298 -> [w479]
          tunnel: w297 -> [w480]
          tunnel: [w477] -> w295
          tunnel: [w476] -> w296
          frame #0 {
            w432 = 0.1 ("Delay Time (s)")
            n223 = property on="Z Step SP" class="DigNum (strict)" props=["Maximum"]() -> ()  [unwired: 2 in, 3 out]
            n224 = call "mDrive Send Command.vi"("error in (no error)"=w426, "Extra"="P", "Command"=T1."Print Parameter", "VISA resource name"=w427) -> ("error out"=w453:errorcluster, "read buffer"=w457:string, "VISA resource name out"=w455:refnum<visa-resource-name>)  [unwired: 3 in]
            n225 = Decimal String To Number(string=w457, offset=0) -> (number=w439:i32)  [unwired: 1 in, 1 out]
            n226 = property on="Z Step SP" class="DigNum (strict)"() -> ("Minimum"=w451:dbl)  [unwired: 2 in, 2 out]
            n227 = property on="Z max step" class="DigNum (strict)"() -> ("Value"=w422:i32)  [unwired: 2 in, 2 out]
            n228 = To Long Integer(number=w439) -> (32bit integer=w440:i32)
            n229 = property on="Z Step PV" class="DigNum (strict)"("Val(Sgnl)"=w440) -> ()  [unwired: 2 in, 2 out]
            n230 = call "Time Delay17"("error in (no error)"=w453, "Delay Time (s)"=w432) -> ("error out"=w452:errorcluster)  [unwired: 9 in]
            n231 = To Long Integer(number=w451) -> (32bit integer=w450:i32)
            n232 = To Long Integer(number=w422) -> (32bit integer=w449:i32)
            n233 = property on="Z steps/rev" class="DigNum (strict)"() -> ("Value"=w446:u32)  [unwired: 2 in, 2 out]
            n234 = To Double Precision Float(number=w446) -> (double precision float=w447:dbl)
            n235 = In Range and Coerce(upper limit=w449, x=w440, lower limit=w450) -> (In Range?=w448:bool)  [unwired: 1 out]
            n236 = To Double Precision Float(number=w440) -> (double precision float=w441:dbl)
            n237 = Divide(x=w441, y=w447) -> (x/y=w445:dbl)
            n238 = property on="APX:MZ_LIM" class="Bool (strict)"("Val(Sgnl)"=w448) -> ()  [unwired: 2 in, 2 out]
            n239 = call "mDrive Send Command.vi"("error in (no error)"=w452, "Extra"="MV", "Command"=T1."Print Parameter", "VISA resource name"=w455) -> ("error out"=w454:errorcluster, "read buffer"=w423:string, "VISA resource name out"=w458:refnum<visa-resource-name>)  [unwired: 3 in]
            n240 = call "Time Delay16"("error in (no error)"=w454, "Delay Time (s)"=w432) -> ("error out"=w437:errorcluster)  [unwired: 9 in]
            n241 = Decimal String To Number(string=w423, offset=0 ("offset (0)")) -> (number=w431:i32)  [unwired: 1 in, 1 out]
            n242 = Not Equal?(x=w423, y="") -> (x != y?=w424:bool)
            n243 = property on="Z mm/rev" class="DigNum (strict)"() -> ("Value"=w444:dbl)  [unwired: 2 in, 2 out]
            n244 = property on="Z offset mm" class="DigNum (strict)"() -> ("Value"=w442:dbl)  [unwired: 2 in, 2 out]
            n245 = Multiply(x=w445, y=w444) -> (x*y=w443:dbl)
            n246 = Number To Boolean Array(number=w431) -> (Boolean array=w430:bool[])
            n247 = property on="APX:MZ_RDY" class="Bool (strict)"("Val(Sgnl)"=w424) -> ()  [unwired: 2 in, 2 out]
            n248 = Add(x=w443, y=w442) -> (x+y=w421:dbl)
            n249 = Index Array(array=w430, index=0) -> (element=w428:bool)
            n250 = property on="APX:MZ_PV" class="DigNum (strict)"("Val(Sgnl)"=w421) -> ()  [unwired: 2 in, 2 out]
            n251 = property on="APX:MZ_MVG" class="Bool (strict)"("Val(Sgnl)"=w428) -> ()  [unwired: 2 in, 2 out]
          }
          frame #1 {
          }
          frame #2 {
            n252 = case shown="True" w464 {
              tunnel: w465 -> [w471 w475]
              tunnel: [w472 w475] -> w466
              tunnel: [w473 w474] -> w467
              tunnel: w468 -> [w470 w474]
              frame False {
                n253 = call "mDrive Send Command.vi"("error in (no error)"=w470, "Command"=T1."Stop", "VISA resource name"=w471) -> ("error out"=w473:errorcluster, "VISA resource name out"=w472:refnum<visa-resource-name>)  [unwired: 4 in, 1 out]
              }
              frame True {
              }
            }
          }
          frame #3 {
            n254 = disable-structure shown="Disabled" {
              disable-tunnel: w480 -> [w486 _]
              disable-tunnel: w479 -> [w484 _]
              disable-tunnel: w478 -> [w483 _]
              disable-tunnel: [w482 _] -> w477
              disable-tunnel: [w481 _] -> w476
              frame Disabled {
                n255 = Implies(1:w486) -> (0:w485:bool, 2:w487:bool)
                n256 = case shown="False" w485 {
                  tunnel: w484 -> [w494 w547]
                  tunnel: w483 -> [w493 w548]
                  tunnel: [w492 w547] -> w482
                  tunnel: [w491 w548] -> w481
                  frame False {
                    # "Backlash"
                    n257 = flat-sequence {
                      tunnel: [w509] -> w506
                      tunnel: [w511] -> w505
                      tunnel: [w510] -> w504
                      tunnel: w494 -> [w508]
                      tunnel: w493 -> [w507]
                      tunnel: w506 -> [w519]
                      tunnel: [w519] -> w503
                      tunnel: w505 -> [w518]
                      tunnel: w504 -> [w517]
                      tunnel: [w516] -> w502
                      tunnel: [w515] -> w501
                      tunnel: [w514] -> w490
                      tunnel: w503 -> [w529]
                      tunnel: w502 -> [w528]
                      tunnel: w501 -> [w526]
                      tunnel: [w527] -> w500
                      tunnel: [w526] -> w499
                      tunnel: [w525] -> w496
                      tunnel: [w524] -> w495
                      tunnel: w490 -> [w524]
                      tunnel: w500 -> [w540]
                      tunnel: w499 -> [w533]
                      tunnel: [w540] -> w498
                      tunnel: [w539] -> w497
                      tunnel: w496 -> [w539]
                      tunnel: w495 -> [w535]
                      tunnel: [w534] -> w488
                      tunnel: w498 -> [w544]
                      tunnel: w497 -> [w543]
                      tunnel: [w542] -> w492
                      tunnel: [w541] -> w489
                      tunnel: w488 -> [w541]
                      tunnel: [w546] -> w491
                      tunnel: w489 -> [w546]
                      frame #0 {
                        n258 = property on="Z Backlash steps/sec" class="DigNum (strict)"() -> ("Value"=w509:i32)  [unwired: 2 in, 2 out]
                        n259 = Number To Decimal String(number=w509) -> (decimal integer string=w512:string)  [unwired: 1 in]
                        n260 = call "mDrive Send Command.vi"("error in (no error)"=w508, "Extra"=w512, "Command"=T1."Max Velocity", "VISA resource name"=w507) -> ("error out"=w510:errorcluster, "VISA resource name out"=w511:refnum<visa-resource-name>)  [unwired: 3 in, 1 out]
                      }
                      frame #1 {
                        n261 = property on="Z Backlash" class="DigNum (strict)"() -> ("Value"=w514:i32)  [unwired: 2 in, 2 out]
                        n262 = Number To Decimal String(number=w514) -> (decimal integer string=w520:string)  [unwired: 1 in]
                        n263 = call "mDrive Send Command.vi"("error in (no error)"=w517, "Extra"=w520, "Command"=T1."Move to Relative Position", "VISA resource name"=w518) -> ("error out"=w516:errorcluster, "VISA resource name out"=w515:refnum<visa-resource-name>)  [unwired: 3 in, 1 out]
                      }
                      frame #2 {
                        n264 = To Double Precision Float(number=w524) -> (double precision float=w522:dbl)
                        n265 = To Double Precision Float(number=w529) -> (double precision float=w531:dbl)
                        n266 = Absolute Value(x=w522) -> (abs(x)=w523:dbl)
                        n267 = Divide(x=w523, y=w531) -> (x/y=w532:dbl)
                        n268 = Add(x=w532, y=0.5) -> (x+y=w525:dbl)
                        n269 = call "Time Delay18"("error in (no error)"=w528, "Delay Time (s)"=w525) -> ("error out"=w527:errorcluster)  [unwired: 9 in]
                      }
                      frame #3 {
                        n270 = Negate(x=w535) -> (-x=w536:i32)
                        n271 = Number To Decimal String(number=w536) -> (decimal integer string=w537:string)  [unwired: 1 in]
                        n272 = call "mDrive Send Command.vi"("Extra"=w537, "Command"=T1."Move to Relative Position", "VISA resource name"=w533) -> ("VISA resource name out"=w534:refnum<visa-resource-name>)  [unwired: 4 in, 2 out]
                      }
                      frame #4 {
                        n273 = call "Time Delay19"("error in (no error)"=w544, "Delay Time (s)"=w543) -> ("error out"=w542:errorcluster)  [unwired: 9 in]
                      }
                      frame #5 {
                        w545 = FALSE ("Value (Signaling)")
                      }
                    }
                  }
                  frame True {
                  }
                }
              }
              frame Enabled {
              }
            }
          }
        }
      }
      event "APX:MZ_RQ": Value Change {
        n274 = event-data() -> ()  [unwired: 1 in, 6 out]
        n275 = property on="APX:MZ_RQ" class="DigNum (strict)"() -> ("Value"=w553:dbl)  [unwired: 2 in, 2 out]
        n276 = property on="APX:MZ_PV" class="DigNum (strict)"() -> ("Value"=w552:dbl)  [unwired: 2 in, 2 out]
        n277 = Less?(x=w553, y=w552) -> (x < y?=w549:bool)
        n278 = property on="Isolated from GND?" class="Bool (strict)"() -> ("Value"=w551:bool)  [unwired: 2 in, 2 out]
        n279 = Or(x=w551, y=w549) -> (x .or. y?=w550:bool)
        n280 = case shown="True" w550 {
          tunnel: w557 -> [w559 w563]
          tunnel: w556 -> [w558 w562]
          tunnel: [w558 w561] -> w555
          tunnel: [w559 w560] -> w554
          frame False {
          }
          frame True {
            n281 = flat-sequence {
              tunnel: w562 -> [w572]
              tunnel: w563 -> [w573]
              tunnel: [w573] -> w571
              tunnel: [w572] -> w570
              tunnel: [w595] -> w569
              tunnel: [w594] -> w568
              tunnel: w571 -> [w597]
              tunnel: w570 -> [w596]
              tunnel: [w613] -> w567
              tunnel: [w612] -> w566
              tunnel: w569 -> [w611]
              tunnel: w568 -> [w610]
              tunnel: [w621] -> w565
              tunnel: [w620] -> w564
              tunnel: w567 -> [w619]
              tunnel: w566 -> [w618]
              tunnel: [w627] -> w561
              tunnel: [w628] -> w560
              tunnel: w565 -> [w628]
              tunnel: w564 -> [w626]
              frame #0 {
                (unwired) T2."Disabled and Grayed Out" ("Disabled")
                (unwired) T2."Disabled and Grayed Out" ("Disabled")
                n282 = flat-sequence {
                  frame #0 {
                    n283 = property on="APX:MZ_RQ" class="DigNum (strict)"() -> ("Value"=w585:dbl)  [unwired: 2 in, 2 out]
                    n284 = property on="Z offset mm" class="DigNum (strict)"() -> ("Value"=w586:dbl)  [unwired: 2 in, 2 out]
                    n285 = property on="APX:MZ_VLC_RQ" class="DigNum (strict)"() -> ("Value"=w579:dbl)  [unwired: 2 in, 2 out]
                    n286 = property on="Z steps/rev" class="DigNum (strict)"() -> ("Value"=w588:u32)  [unwired: 2 in, 2 out]
                    n287 = property on="Z mm/rev" class="DigNum (strict)"() -> ("Value"=w591:dbl)  [unwired: 2 in, 2 out]
                    n288 = Subtract(x=w585, y=w586) -> (x-y=w589:dbl)
                    n289 = property on="Z Velocity SP step/sec" class="DigNum (strict)"() -> ("Maximum"=w575:dbl)  [unwired: 2 in, 2 out]
                    n290 = property on="Z Velocity SP step/sec" class="DigNum (strict)"() -> ("Minimum"=w574:dbl)  [unwired: 2 in, 2 out]
                    n291 = Divide(x=w579, y=w591) -> (x/y=w580:dbl)
                    n292 = Divide(x=w589, y=w591) -> (x/y=w590:dbl)
                    n293 = To Double Precision Float(number=w588) -> (double precision float=w592:dbl)
                    n294 = property on="Z Step SP" class="DigNum (strict)"() -> ("Maximum"=w582:dbl)  [unwired: 2 in, 2 out]
                    n295 = property on="Z Step SP" class="DigNum (strict)"() -> ("Minimum"=w581:dbl)  [unwired: 2 in, 2 out]
                    n296 = Multiply(x=w580, y=w592) -> (x*y=w577:dbl)
                    n297 = Multiply(x=w590, y=w592) -> (x*y=w584:dbl)
                    n298 = In Range and Coerce(upper limit=w575, x=w577, lower limit=w574) -> (coerced(x)=w576:dbl)  [unwired: 1 out]
                    n299 = In Range and Coerce(upper limit=w582, x=w584, lower limit=w581) -> (coerced(x)=w583:dbl)  [unwired: 1 out]
                    n300 = To Long Integer(number=w576) -> (32bit integer=w578:i32)
                    n301 = To Long Integer(number=w583) -> (32bit integer=w587:i32)
                    n302 = property on="Z Velocity SP step/sec" class="DigNum (strict)"("Val(Sgnl)"=w578) -> ()  [unwired: 2 in, 2 out]
                    n303 = property on="Z Step SP" class="DigNum (strict)"("Val(Sgnl)"=w587) -> ()  [unwired: 2 in, 2 out]
                  }
                }
              }
              frame #1 {
                n304 = property on="Z Step SP" class="DigNum (strict)"() -> ("Value"=w605:i32)  [unwired: 2 in, 2 out]
                n305 = property on="Z Step PV" class="DigNum (strict)"() -> ("Value"=w604:i32)  [unwired: 2 in, 2 out]
                n306 = property on="Z Backlash" class="DigNum (strict)"() -> ("Value"=w593:i32)  [unwired: 2 in, 2 out]
                n307 = Subtract(x=w605, y=w604) -> (x-y=w603:i32)
                n308 = Sign(1:w603) -> (0:w602:i32)
                n309 = Sign(1:w593) -> (0:w601:i32)
                n310 = Multiply(x=w602, y=w601) -> (x*y=w600:i32)
                n311 = Equal?(x=w600, y=1) -> (x = y?=w598:bool)
                n312 = case shown="True" w598 {
                  tunnel: w597 -> [w607 w609]
                  tunnel: w596 -> [w606 w608]
                  tunnel: [w606 w608] -> w595
                  tunnel: [w607 w609] -> w594
                  frame False {
                    (unwired) FALSE ("Value (Signaling)")
                  }
                  frame True {
                    (unwired) TRUE ("Value (Signaling)")
                  }
                }
              }
              frame #2 {
                # "Velocity Setting"
                n313 = property on="Z Velocity SP step/sec" class="DigNum (strict)"() -> ("Value"=w614:i32)  [unwired: 2 in, 2 out]
                n314 = Number To Decimal String(number=w614) -> (decimal integer string=w615:string)  [unwired: 1 in]
                n315 = call "mDrive Send Command.vi"("error in (no error)"=w611, "Extra"=w615, "Command"=T1."Max Velocity", "VISA resource name"=w610) -> ("error out"=w612:errorcluster, "VISA resource name out"=w613:refnum<visa-resource-name>)  [unwired: 3 in, 1 out]
              }
              frame #3 {
                # "Move to Abs Position"
                n316 = call "Time Delay7"("error in (no error)"=w618) -> ("error out"=w617:errorcluster)  [unwired: 10 in]
                n317 = property on="Z Step SP" class="DigNum (strict)"() -> ("Value"=w624:i32)  [unwired: 2 in, 2 out]
                n318 = Number To Decimal String(number=w624) -> (decimal integer string=w623:string)  [unwired: 1 in]
                n319 = call "mDrive Send Command.vi"("error in (no error)"=w617, "Extra"=w623, "Command"=T1."Move to Absolute Position", "VISA resource name"=w619) -> ("error out"=w620:errorcluster, "VISA resource name out"=w621:refnum<visa-resource-name>)  [unwired: 3 in, 1 out]
              }
              frame #4 {
                n320 = call "Time Delay28"("error in (no error)"=w626, "Delay Time (s)"=0.1) -> ("error out"=w627:errorcluster)  [unwired: 9 in]
              }
            }
          }
        }
      }
    }
  }
  n321 = flat-sequence {
    tunnel: w21 -> [w635]
    tunnel: w20 -> [w633]
    tunnel: [w630] -> w19
    frame #0 {
      n322 = call "mDrive Send Command.vi"("error in (no error)"=w633, "Extra"="P", "Command"=T1."Print Parameter", "VISA resource name"=w635) -> ("error out"=w632:errorcluster, "read buffer"=w639:string, "VISA resource name out"=w634:refnum<visa-resource-name>)  [unwired: 3 in]
      n323 = call "Time Delay32"("error in (no error)"=w632) -> ("error out"=w629:errorcluster)  [unwired: 10 in]
      n324 = Decimal String To Number(string=w639, offset=0) -> (number=w631:i32)  [unwired: 1 in, 1 out]
      n325 = To Long Integer(number=w631) -> (32bit integer=w630:i32)
      n326 = call "mDrive Send Command.vi"("error in (no error)"=w629, "Command"=T1."Stop", "VISA resource name"=w634) -> ("error out"=w641:errorcluster, "VISA resource name out"=w642:refnum<visa-resource-name>)  [unwired: 4 in, 1 out]
      n327 = VISA Close(VISA resource name=w642, error in (no error)=w641) -> ()  [unwired: 1 out]
    }
  }
  n328 = flat-sequence {
    tunnel: w19 -> [w648]
    frame #0 {
      n329 = Build Array(0 ("element"), 0 ("element"), w648, 0 ("element")) -> (w646:i32[])
      n330 = call-poly <vilib>:"Write To Spreadsheet File.vi"("1D data"=w646, "file path (dialog if empty)"=path "S:/SSE/IMS/POSZ.TXT") -> ()  [unwired: 6 in, 1 out]
    }
    frame #1 {
    }
  }
